vi "Write Value Source.vi"(8 "error in (no error)":errorcluster, 10 "Value Source":refnum<class "Value Source.lvclass">, 11 "Composed Column in":refnum<class "Composed Column.lvclass">) -> (0 "error out":errorcluster, 3 "Composed Column out":refnum<class "Composed Column.lvclass">)   [LabVIEW 2020, in "Composed Columns.lvlib" / "Composed Column.lvclass"]
uses:
  Composed Column.lvclass
  Composed Columns/Value Source Interface Class/Value Source.lvclass
  Composed Column.lvclass/Composed Column.ctl
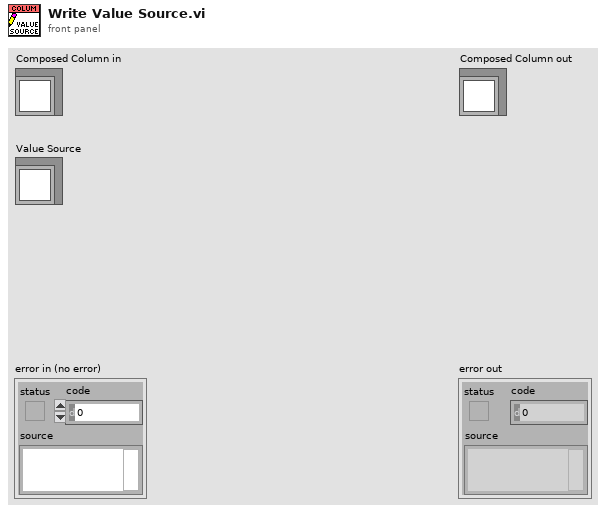
[diagram p1: front panel]
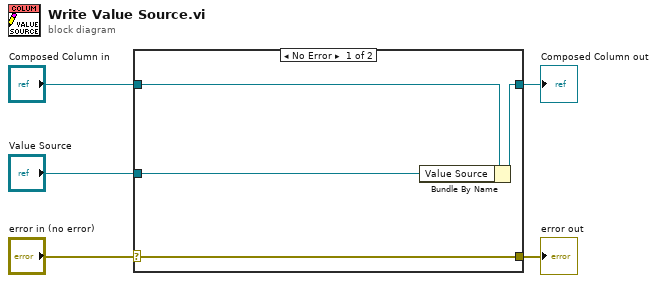
[diagram p0: block diagram]
diagram:
  n1 = case shown="No Error" "error in (no error)" {
    selector: "error in (no error)" -> [w9 w10]
    tunnel: [w9 w10] -> w4
    tunnel: [w7 w11] -> w2
    tunnel: "Composed Column in" -> [w8 w11]
    tunnel: "Value Source" -> [w6 _]
    frame No Error {
      n2 = Bundle By Name(cluster=w8, "Value Source"=w6) -> (w7:refnum<class "Composed Column.lvclass">)
    }
    frame Error {
    }
  }
  "error out" <- w4
  "Composed Column out" <- w2
